vi "API - ADC - Enable Analog Input Channel.vi"(8 "error in (no error)":errorcluster, 10 "Analog Input Channel Number":i32, 11 "DAQiFi Device Properties In":T1) -> (0 "error out":errorcluster, 3 "DAQiFi Device Properties Out":T1)   [LabVIEW 2021]
doc: "Send a command to the DAQ which enables an analog input channel."
uses:
  TypeDefs/TypeDef - Cluster of DAQiFi Device Properties.ctl
  TypeDefs/Enum - Connection Type.ctl
  TCP - Write and Read a Synchronous Message.vi
  USB - Write and Read a Synchronous Message.vi
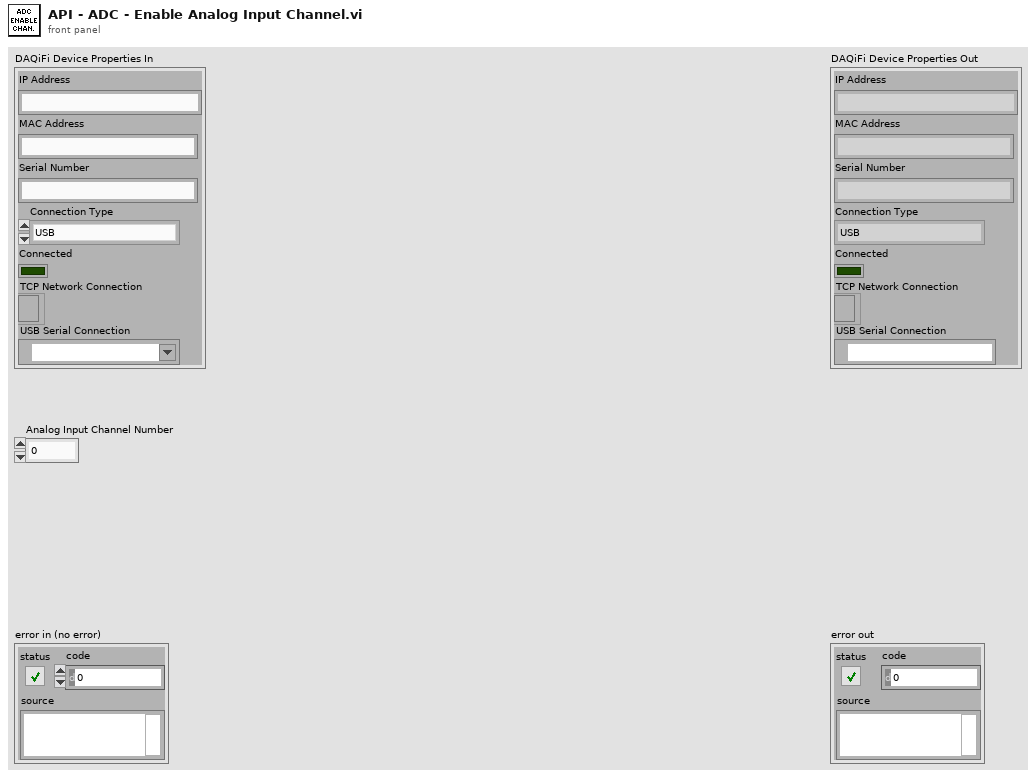
[diagram p1: front panel]
types:
  T1 = typedef "TypeDef - Cluster of DAQiFi Device Properties.ctl" = cluster{"IP Address":string, "MAC Address":string, "Serial Number":string, "Connection Type":T2, "Connected":bool, "TCP Network Connection":refnum<k5>, "USB Serial Connection":refnum<visa-resource-name>}
  T2 = typedef "Enum - Connection Type.ctl" = enum16{"USB", "TCP"}
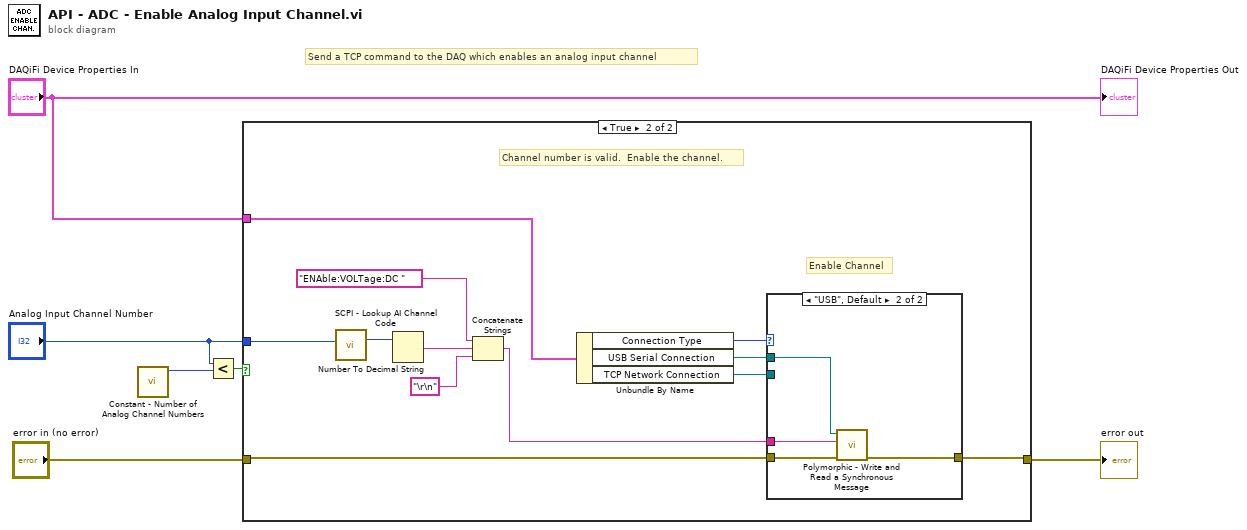
[diagram p0: block diagram]
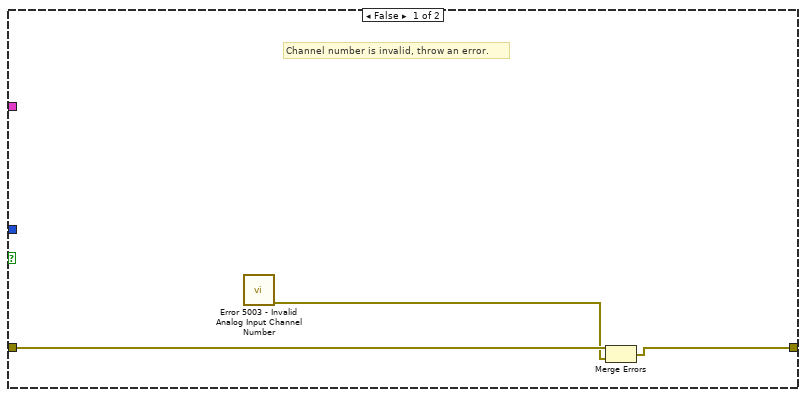
[diagram p2: hidden frame]
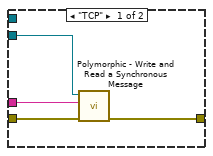
[diagram p3: hidden frame]
diagram:
  # "Send a TCP command to the DAQ which enables an analog input channel"
  n1 = call "Constant - Number of Analog Channel Numbers.vi"() -> ("Maximum Channel"=w3:i32)  [unwired: 11 in]
  n2 = Less?(x="Analog Input Channel Number", y=w3) -> (x < y?=w2:bool)
  n3 = case shown="True" w2 {
    tunnel: [w8 w15] -> w6
    tunnel: "error in (no error)" -> [w9 w16]
    tunnel: "Analog Input Channel Number" -> [_ w17]
    tunnel: "DAQiFi Device Properties In" -> [_ w14]
    frame False {
      # "Channel number is invalid, throw an error."
      n4 = call "Error 5003 - Invalid Analog Input Channel Number.vi"() -> ("error out"=w7:errorcluster)  [unwired: 11 in]
      n5 = Merge Errors(w9, w7) -> (w8:errorcluster)
    }
    frame True {
      # "Channel number is valid.  Enable the channel."
      # "Enable Channel"
      n6 = call "SCPI - Lookup AI Channel Code.vi"("Analog Input Channel Number"=w17) -> ("Channel Code"=w18:i32)  [unwired: 10 in]
      n7 = Number To Decimal String(number=w18) -> (decimal integer string=w20:string)  [unwired: 1 in]
      n8 = Concatenate Strings("ENAble:VOLTage:DC " ("Message to Send"), w20, "\r\n" ("string")) -> (w12:string)
      n9 = Unbundle By Name(w14) -> ("Connection Type"=w13:T2, "USB Serial Connection"=w10:refnum<visa-resource-name>, "TCP Network Connection"=w11:refnum<k5>)
      n10 = case shown="\"USB\", Default" w13 {
        tunnel: w16 -> [w25 w29]
        tunnel: [w24 w28] -> w15
        tunnel: w12 -> [w23 w27]
        tunnel: w11 -> [w22 _]
        tunnel: w10 -> [_ w26]
        frame "TCP" {
          n11 = call-poly "Polymorphic - Write and Read a Synchronous Message.vi"("error in"=w25, "Message to Send"=w23, "TCP Network Connection in"=w22) -> ("error out"=w24:errorcluster)  [unwired: 6 in, 2 out]
        }
        frame "USB", Default {
          n12 = call-poly "Polymorphic - Write and Read a Synchronous Message.vi"("error in"=w29, "Message to Send"=w27, "VISA resource name in"=w26) -> ("error out"=w28:errorcluster)  [unwired: 6 in, 2 out]
        }
      }
    }
  }
  "error out" <- w6
  "DAQiFi Device Properties Out" <- "DAQiFi Device Properties In"
